vi "ma_Force Restart.vi"(6 "caller VI name":string, 7 "force restart averaging in":bool, 8 "linear averaging done":bool, 9 "restart averaging (F)":bool, 10 "window":T2=1 items=["Rectangle"=0, "Hanning"=1, "Hamming"=2, "Blackman-Harris"=3, "Exact Blackman"=4, "Blackman"=5, "Flat Top"=6, "4 Term B-Harris "=7, "7 Term B-Harris"=8, "Low Sidelobe"=9, "Blackman Nuttall"=11, "Triangle"=30, "Bartlett-Hanning"=31, "Bohman"=32, "Parzen"=33, "Welch"=34, "Kaiser"=60, "Dolph-Chebyshev"=61, "Gaussian"=62], 11 "averaging parameters":T1={"averaging mode"=enum."No averaging", "weighting mode"=enum."Exponential", "number of averages"=10} {"number of averages" min=1}) -> (0 "error out":errorcluster, 1 "retrieve last spectrum":bool, 2 "force restart averaging":bool, 3 "skip processing":errorcluster)   [LabVIEW 2020, in "NI_MAPro.lvlib"]
uses:
  NI_MAPro.lvlib
  windowTd.ctl
  NI_AALPro.lvlib
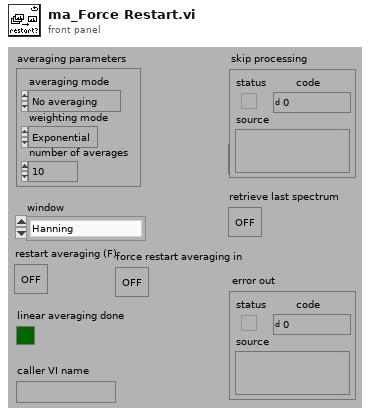
[diagram p1: front panel]
types:
  T1 = cluster{"averaging mode":enum16{"No averaging", "Vector averaging", "RMS averaging", "Peak hold"}, "weighting mode":enum16{"Linear", "Exponential"}, "number of averages":u32}
  T2 = typedef "NI_AALPro.lvlib/windowTd.ctl" = u32
  T3 = enum16{"No averaging", "Vector averaging", "RMS averaging", "Peak hold"}
  T4 = cluster{"averaging parameters":cluster{"averaging mode":enum16{"No averaging", "Vector averaging", "RMS averaging", "Peak hold"}, "weighting mode":enum16{"Linear", "Exponential"}, "number of averages":u32}, "window":T2}
  T5 = cluster{"status":bool, "code":i32, "caller VI name":string}
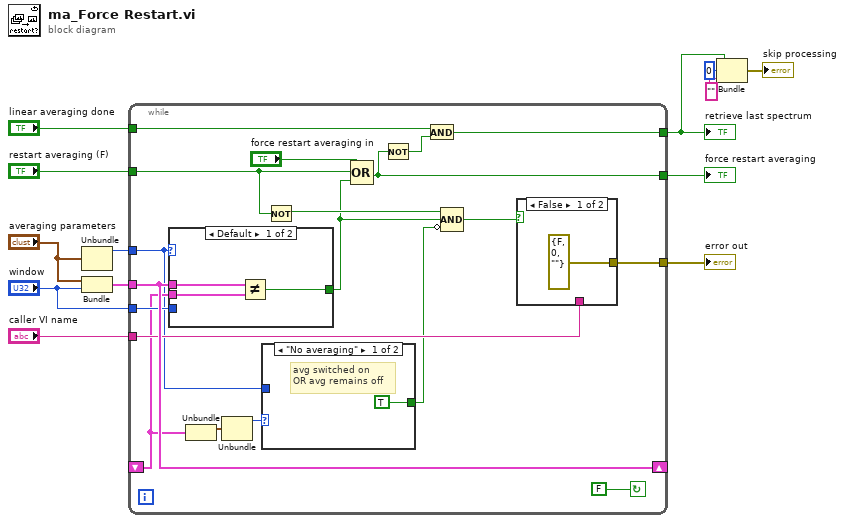
[diagram p0: block diagram]
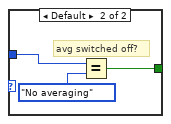
[diagram p2: hidden frame]
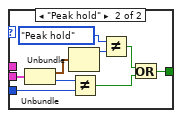
[diagram p3: hidden frame]
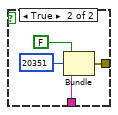
[diagram p4: hidden frame]
diagram:
  n1 = Unbundle("averaging parameters") -> ("averaging mode"=w4:T3)  [unwired: 2 out]
  n2 = Bundle("averaging parameters"="averaging parameters", "window"="window") -> (w2:T4)  [unwired: 1 out]
  n3 = while {
    tunnel: "window" -> [w26]
    tunnel: w2 -> [w27]
    tunnel: w4 -> [w14]
    tunnel: "caller VI name" -> [w18]
    tunnel: [w28] -> w6
    shift-left: _ -> [w17]
    shift-right: [w27] -> _
    tunnel: [w32] -> w7
    tunnel: [w24] -> w11
    tunnel: "linear averaging done" -> [w30]
    tunnel: "restart averaging (F)" -> [w25]
    stop <- FALSE continue-if-true
    n4 = case shown="Default" w14 {
      tunnel: w17 -> [w39 w48]
      tunnel: [w38 w42] -> w21
      tunnel: w27 -> [w37 _]
      tunnel: w26 -> [_ w46]
      frame Default {
        n5 = Not Equal?(x=w37, y=w39) -> (x != y?=w38:bool)
      }
      frame "Peak hold" {
        n6 = Unbundle(w48) -> ("averaging parameters"=w45:T1, "window"=w47:T2)
        n7 = Unbundle(w45) -> ("averaging mode"=w41:T3)  [unwired: 2 out]
        n8 = Not Equal?(x=w47, y=w46) -> (x != y?=w43:bool)
        n9 = Not Equal?(x=T3."Peak hold" ("y"), y=w41) -> (x != y?=w44:bool)
        n10 = Or(x=w44, y=w43) -> (x .or. y?=w42:bool)
      }
    }
    n11 = Unbundle(w17) -> ("averaging parameters"=w19:T1)  [unwired: 1 out]
    n12 = Unbundle(w19) -> ("averaging mode"=w15:T3)  [unwired: 2 out]
    n13 = case shown="\"No averaging\"" w15 {
      tunnel: w14 -> [_ w36]
      tunnel: [TRUE w34] -> w16
      frame "No averaging" {
        # "avg switched on \nOR avg remains off"
      }
      frame Default {
        # "avg switched off?"
        n14 = Equal?(x=w36, y=T3."No averaging" ("averaging mode")) -> (x = y?=w34:bool)
      }
    }
    n15 = Not(x=w25) -> (.not. x?=w22:bool)
    n16 = Compound Arithmetic op=OR("force restart averaging in", w25, w21) -> (w24:bool)
    n17 = Not(x=w24) -> (.not. x?=w29:bool)
    n18 = And(x=w30, y=w29) -> (x .and. y?=w32:bool)
    n19 = Compound Arithmetic op=AND(w22, w21, invert w16) -> (w20:bool)
    n20 = case shown="False" w20 {
      tunnel: [errorcluster {"status"=FALSE, "code"=0, "source"=""} ("error out") w53] -> w28
      tunnel: w18 -> [_ w50]
      frame False {
      }
      frame True {
        n21 = Bundle("status"=FALSE, "code"=20351, "caller VI name"=w50) -> (w53:T5)  [unwired: 1 out]
      }
    }
  }
  "force restart averaging" <- w11
  "retrieve last spectrum" <- w7
  "error out" <- w6
  n22 = Bundle(w7, "code"=0, "source"="") -> (→"skip processing":cluster{bool, "code":i32, "source":string})  [unwired: 1 out]
